vi "Notebook Shortcuts.vi"() -> ()   [LabVIEW 2019, in "Notebook.lvlib"]
uses:
  Notebook.lvlib
panel:
  out "String":string="Notebook Useful Keyboard Shortcuts\n\nCtrl+Tab                               Tab\t\nCtrl+A                                   Select all\t\nCtrl+E                                   Center alignment\t\nCtrl+J                                    Justify alignment\t\nCtrl+R                                   Right alignment\t\nCtrl+L                                  \tLeft alignment\t\nCtrl+C\t                                 Copy\t\nCtrl+V\t                                  Paste\t\nCtrl+X\t                                  Cut\t\nCtrl+Z\t                                  Undo\t\nCtrl+Y\t                                  Redo\t\nCtrl+'+' (Ctrl+Shift+'=')\t    Superscript\t\nCtrl+'='\t                                Subscript\t\nCtrl+1\t                                   Line spacing = 1 line.\t\nCtrl+2\t                                   Line spacing = 2 lines.\t\nCtrl+5\t                                   Line spacing = 1.5 lines.\t\nCtrl+' (apostrophe)\t            Accent acute\nCtrl+` (grave)\t                      Accent grave\nCtrl+~ (tilde)\t                       Accent tilde\nCtrl+; (semicolon)\t              Accent umlaut\nCtrl+Shift+6\t                        Accent caret (circumflex)\nCtrl+, (comma)\t                  Accent cedilla\nCtrl+Shift+' (apostrophe)\t Activate smart quotes\t\nCtrl+Backspace\t                  Delete previous word.\nCtrl+Left Arrow\t                  Move cursor one word to the left.\nCtrl+Right Arrow\t                Move cursor one word to the right\nCtrl+Left Shift                      Left alignment\nCtrl+Right Shift\t                  Right alignment\nCtrl+Up Arrow\t                    Move to the line above.\nCtrl+Down Arrow\t               Move to the line below.\nCtrl+Home\t                          Move to the beginning of the document\nCtrl+End\t                              Move to the end of the document.\nCtrl+Page Up\t                      Move one page up\nCtrl+Page Down\t                 Move one page down\nCtrl+Delete\t                          Delete the next word or selected characters\nShift+Delete\t                        Cut the selected characters.\t\nCtrl+Shift+A\t                        Set all caps.\t\nCtrl+Shift+L\t                         Fiddle bullet style.\t\nCtrl+Shift+Right Arrow\t      Increase font size\nCtrl+Shift+Left Arrow\t         Decrease font size"
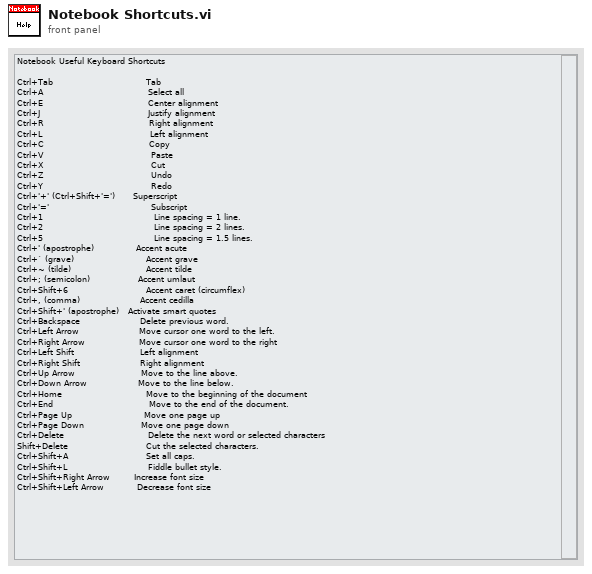
[diagram p1: front panel]
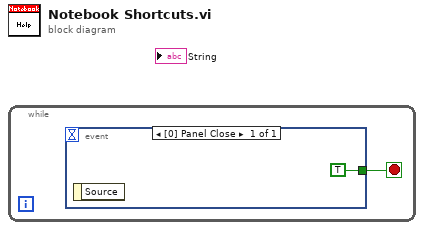
[diagram p0: block diagram]
diagram:
  n1 = while {
    stop <- w1 stop-if-true
    n2 = event shown="[0] Panel Close" {
      selector: _ -> [_]
      dyn-events: _ -> [_]
      timeout: _ -> [_]
      tunnel: [TRUE] -> w1
      event Panel Close {
        n3 = event-data() -> ()  [unwired: 1 in, 1 out]
      }
    }
  }
